vi "clone.vi"(0 "reference":refnum<class "SystemNode.lvclass">, 5 "error in (no error)":errorcluster) -> (14 "reference out":refnum<class "SystemNode.lvclass">, 15 "clonedPackageNode":refnum<class "AbstractNode.lvclass">, 19 "error out":errorcluster)   [LabVIEW 2020, in "SystemNode.lvclass"]
doc: "public Object clone()"
uses:
  <resource>/Framework/Providers/Open_GDS/UML/SystemNode_class/SystemNode.lvclass
  C:/Program Files (x86)/National Instruments/LabVIEW 2020/resource/Framework/Providers/Open_GDS/UML/RectangularNode_class/RectangularNode.lvclass
  C:/Program Files (x86)/National Instruments/LabVIEW 2020/resource/Framework/Providers/Open_GDS/UML/AbstractNode_class/AbstractNode.lvclass
  <resource>/Framework/Providers/Open_GDS/UML/AbstractNode_class/AbstractNode.lvclass
  <resource>/Framework/Providers/Open_GDS/UML/MultiLineString_class/MultiLineString.lvclass
  <resource>/Framework/Providers/Open_GDS/UML/RectangularNode_class/RectangularNode.lvclass
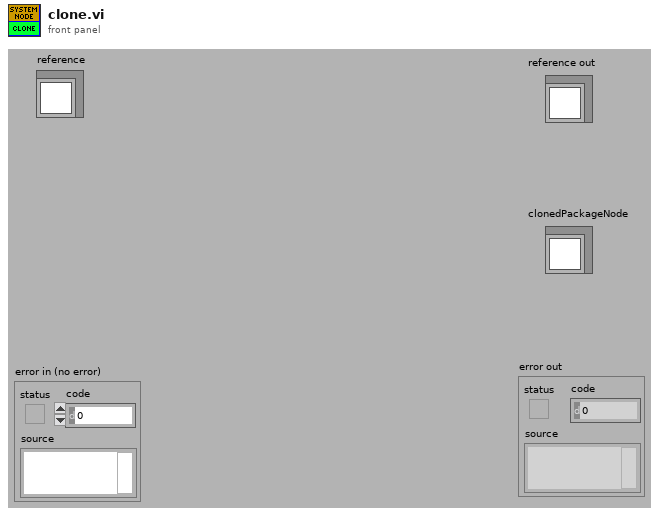
[diagram p1: front panel]
types:
  T1 = typedef "SystemNode.lvclass/ObjectAttributes.ctl" = cluster{"contents":refnum<class "MultiLineString.lvclass">, "DEFAULT_WIDTH":i32, "DEFAULT_HEIGHT":i32, "NAME_GAP":i32, "XGAP":i32, "YGAP":i32}
  T2 = typedef "RectangularNode.lvclass/ObjectAttributes.ctl" = cluster{"bounds":T3}
  T3 = typedef "Rectangle Rectangle2D.ctl" = cluster{"x":dbl, "y":dbl, "width":dbl, "height":dbl}
  T4 = typedef "AbstractNode.lvclass/ObjectAttributes.ctl" = cluster{"parent":refnum<class "AbstractNode.lvclass">, "children":refnum<class "AbstractNode.lvclass">[], "Hidden":bool}
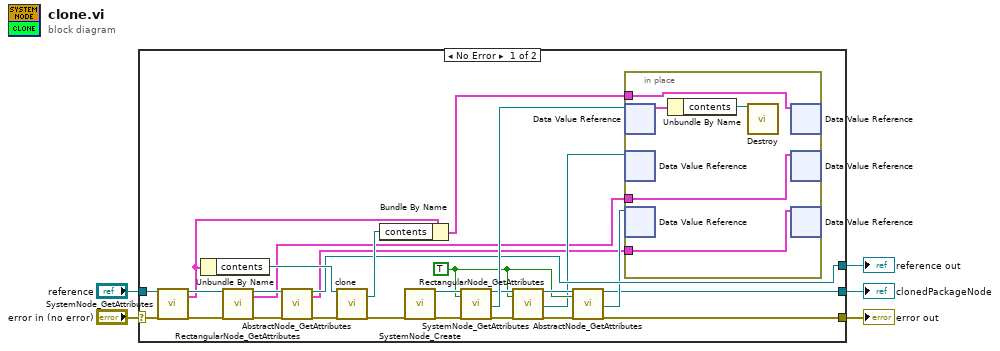
[diagram p0: block diagram]
diagram:
  n1 = case shown="No Error" "error in (no error)" {
    selector: "error in (no error)" -> [w31 w38]
    tunnel: "reference" -> [w32 w39]
    tunnel: [w9 w38] -> w4
    tunnel: [w20 w39] -> w3
    tunnel: [w8 _] -> w1
    frame No Error {
      w12 = TRUE ("OnlyGetDvrReference(False)")
      n2 = call <resource>:"SystemNode_GetAttributes.vi"("reference in"=w32, "error in (no error)"=w31) -> ("reference out"=w26:refnum<class "SystemNode.lvclass">, "Data"=w24:T1, "error out"=w18:errorcluster)  [unwired: 1 in, 14 out]
      n3 = Unbundle By Name(w24) -> ("contents"=w30:refnum<class "MultiLineString.lvclass">)
      n4 = call <resource>:"RectangularNode_GetAttributes.vi"("reference in"=w26, "error in (no error)"=w18) -> ("reference out"=w21:refnum<class "SystemNode.lvclass">, "Data"=w7:T2, "error out"=w19:errorcluster)  [unwired: 14 in, 1 out]
      n5 = call <resource>:"AbstractNode_GetAttributes.vi"("reference in"=w21, "error in (no error)"=w19) -> ("reference out"=w20:refnum<class "SystemNode.lvclass">, "Data"=w6:T4, "error out"=w17:errorcluster)  [unwired: 14 in, 1 out]
      n6 = call-dynamic "clone.vi"("reference"=w30, "error in (no error)"=w17) -> ("clonedMultiLineString"=w23:refnum<class "MultiLineString.lvclass">, "error out"=w27:errorcluster)  [unwired: 15 in, 1 out]
      n7 = Bundle By Name(cluster=w24, "contents"=w23) -> (w22:T1)
      n8 = call <resource>:"SystemNode_Create.vi"("error in (no error)"=w27) -> ("reference out"=w28:refnum<class "SystemNode.lvclass">, "error out"=w29:errorcluster)  [unwired: 17 in]
      n9 = call <resource>:"SystemNode_GetAttributes.vi"("reference in"=w28, "OnlyGetDvrReference(False)"=w12, "error in (no error)"=w29) -> ("reference out"=w14:refnum<class "SystemNode.lvclass">, "DataRef"=w25:refnum<data-value>, "error out"=w15:errorcluster)  [unwired: 13 in, 1 out]
      n10 = call <resource>:"RectangularNode_GetAttributes.vi"("reference in"=w14, "OnlyGetDvrReference(False)"=w12, "error in (no error)"=w15) -> ("reference out"=w13:refnum<class "SystemNode.lvclass">, "DataRef"=w11:refnum<data-value>, "error out"=w16:errorcluster)  [unwired: 13 in, 1 out]
      n11 = call <resource>:"AbstractNode_GetAttributes.vi"("reference in"=w13, "OnlyGetDvrReference(False)"=w12, "error in (no error)"=w16) -> ("reference out"=w8:refnum<class "SystemNode.lvclass">, "DataRef"=w10:refnum<data-value>, "error out"=w9:errorcluster)  [unwired: 13 in, 1 out]
      n12 = in-place {
        in-place-border: w22 -> [w37]
        in-place-border: w7 -> [w36]
        in-place-border: w6 -> [w35]
        n13 = in-place-dvr #1(w25) -> (w33:T1)  [unwired: 1 out]
        n14 = in-place-dvr #2(w11) -> ()  [unwired: 2 out]
        n15 = in-place-dvr #3(w10) -> ()  [unwired: 2 out]
        n16 = Unbundle By Name(w33) -> ("contents"=w34:refnum<class "MultiLineString.lvclass">)
        n17 = call-dynamic "Destroy.vi"("reference"=w34) -> ()  [unwired: 17 in, 2 out]
        n18 = in-place-dvr #1(w37) -> ()  [unwired: 2 out]
        n19 = in-place-dvr #2(w36) -> ()  [unwired: 2 out]
        n20 = in-place-dvr #3(w35) -> ()  [unwired: 2 out]
      }
    }
    frame Error {
    }
  }
  "reference out" <- w3
  "error out" <- w4
  "clonedPackageNode" <- w1
